vi "Capture.vi"(9 "force_length":i8, 10 "capture_channel":u16, 11 "length":i32) -> (3 "function return":i32)   [LabVIEW 2021, in "vmmso.lvlib"]
doc: "DLL_API int WINAPI Capture(int length, unsigned short capture_channel, char force_length);"
uses:
  vmmso.lvlib
  vmmso.dll
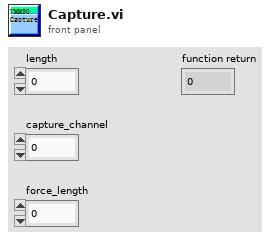
[diagram p1: front panel]
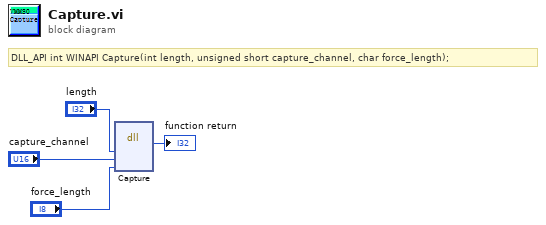
[diagram p0: block diagram]
diagram:
  # "DLL_API int WINAPI Capture(int length, unsigned short capture_channel, char force_length);"
  n1 = dll-call lib="D:/labviewdemo/LabviewDemo 21/vmmso/vmmso.*" fn="Capture"("length"="length", "capture_channel"="capture_channel", "force_length"="force_length") -> (→"function return":i32)  [unwired: 6 in, 2 out]
